vi "BRig_dataBlock_c_BTPR_L.vi"() -> (2 "output_c_BTPR_L":i32)   [LabVIEW 2014]
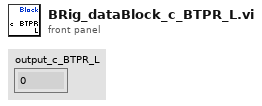
[diagram p1: front panel]
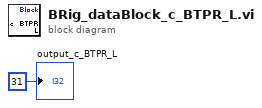
[diagram p0: block diagram]
diagram:
  "output_c_BTPR_L" <- 31 ("output_iBlock")
